vi "Arduino Microcontrollers.vi"   [LabVIEW 2011]
uses:
  _GlobalVariables&Libraries/ATV Program Global Variables.vi
  <vilib>/LabVIEW Interface for Arduino/LabVIEW Interface for Arduino.lvlib
types:
  T1 = cluster{"Arduino 1 VISA resource":refnum<visa-resource-name>, "Front Right Sonar Analog In Voltage":dbl, "Front Left Sonar Analog In Voltage":dbl, "Disable Arduino 1":bool}
  T2 = cluster{"Arduino 2 VISA resource":refnum<visa-resource-name>, "Front Center I2C Data":u8[], "Disable Arduino 2":bool, "Rear Left I2C Data":u8[], "Rear Right I2C Data":u8[]}
  T3 = typedef "LabVIEW Interface for Arduino.lvlib/Arduino Resource.ctl" = cluster{"VISA resource":refnum<visa-resource-name>, "Board Type":T4, "Connection Type":enum8{"USB / Serial"}, "Bytes Per Packet (15)":u8}
  T4 = typedef "LabVIEW Interface for Arduino.lvlib/Board Type.ctl" = enum16{"Uno", "Dimuelanove w/Atmega 328", "Mega 2560"}
  T5 = cluster{"Obstacle Detected":bool, "Drive Speed":string, "Steer Angle":string, "Left Object":bool, "Right Object":bool, "Center Object":bool, "Rear Left":bool, "Rear Right":bool}
  T6 = cluster{"End ATV Program":bool, "E-Stop":bool, "Save Logfile":bool, "Logfile Iteration Delay (ms)":u32, "Loop iteration time (ms)":u32, "Logfile Location":path, "Default GPS Navigation Path":path, "Computer":string, "Default GPS Boundary Path":path}
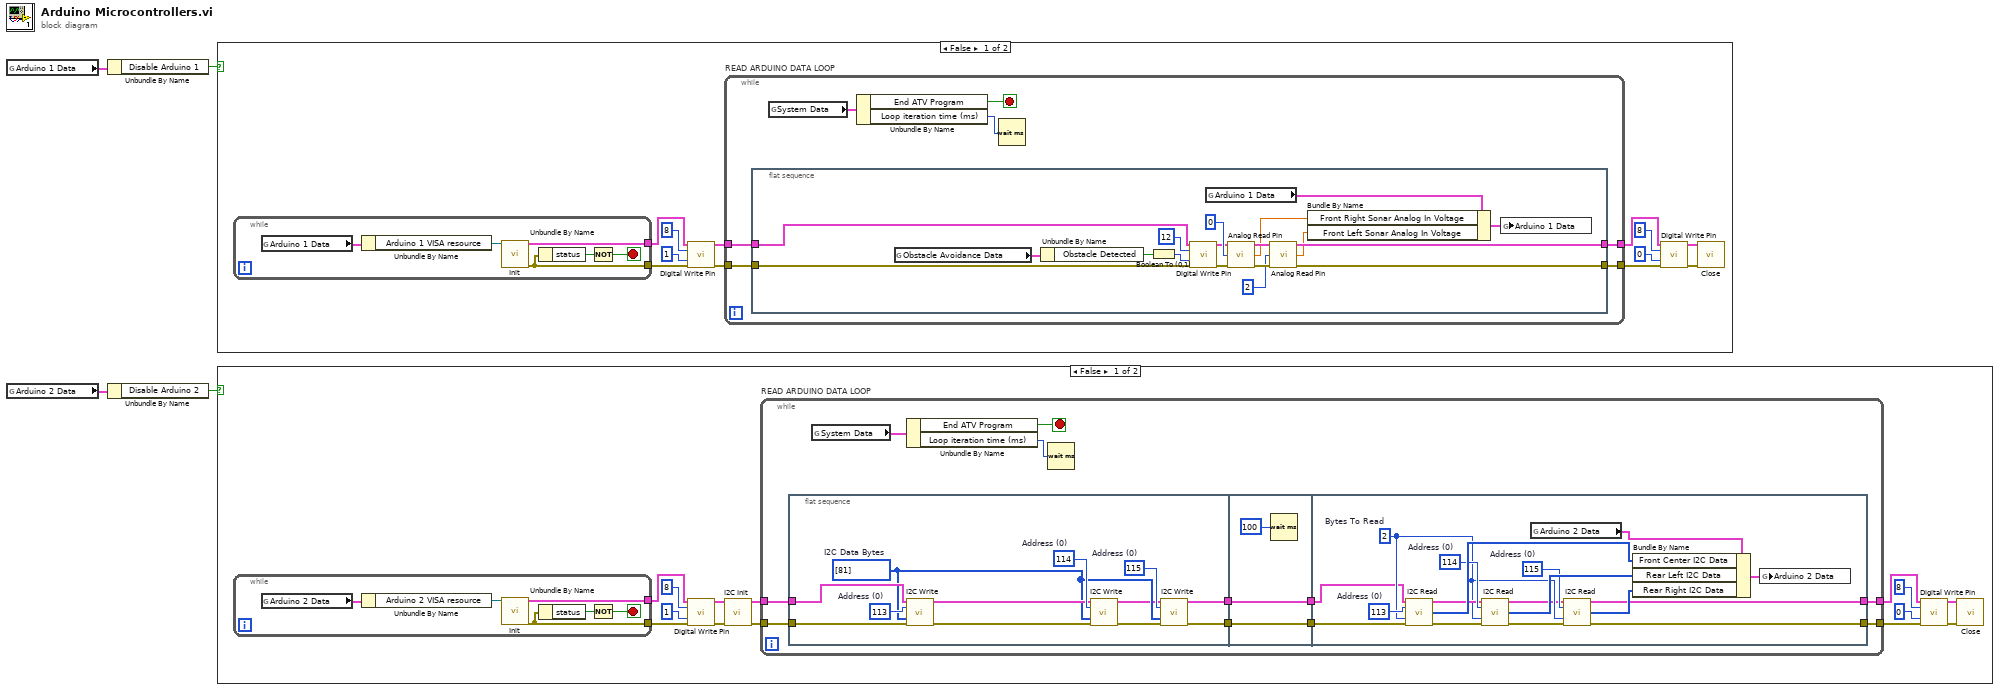
[diagram p0: block diagram]
diagram:
  n1 = global read "ATV Program Global Variables.vi" "Arduino 1 Data"() -> (w4:T1)
  n2 = global read "ATV Program Global Variables.vi" "Arduino 2 Data"() -> (w2:T2)
  n3 = Unbundle By Name(w4) -> ("Disable Arduino 1"=w3:bool)
  n4 = Unbundle By Name(w2) -> ("Disable Arduino 2"=w1:bool)
  n5 = case shown="False" w3 {
    frame False {
      n6 = while {
        tunnel: [w22] -> w16
        tunnel: [w21] -> w15
        stop <- w17 stop-if-true
        n7 = global read "ATV Program Global Variables.vi" "Arduino 1 Data"() -> (w20:T1)
        n8 = Unbundle By Name(w20) -> ("Arduino 1 VISA resource"=w19:refnum<visa-resource-name>)
        n9 = call <vilib>:"Init.vi"("VISA resource"=w19) -> ("Arduino Resource"=w22:T3, "error out"=w21:errorcluster)  [unwired: 17 in]
        n10 = Unbundle By Name(w21) -> ("status"=w18:bool)
        n11 = Not(x=w18) -> (.not. x?=w17:bool)
      }
      n12 = call <vilib>:"Digital Write Pin.vi"("Arduino Resource"=w16, "Digital I/O Pin (0)"=u8 8, "Value (0)"=u8 1, "error in"=w15) -> ("Arduino Resource"=w14:T3, "error out"=w13:errorcluster)  [unwired: 10 in]
      n13 = while "READ ARDUINO DATA LOOP" {
        tunnel: [w29] -> w10
        tunnel: [w28] -> w9
        tunnel: w14 -> [w24]
        tunnel: w13 -> [w23]
        stop <- w26 stop-if-true
        n14 = flat-sequence {
          tunnel: [w44] -> w28
          tunnel: [w45] -> w29
          tunnel: w24 -> [w35]
          tunnel: w23 -> [w34]
          frame #0 {
            n15 = global read "ATV Program Global Variables.vi" "Obstacle Avoidance Data"() -> (w31:T5)
            n16 = Unbundle By Name(w31) -> ("Obstacle Detected"=w30:bool)
            n17 = Boolean To (0,1)(Boolean=w30) -> (0, 1=w37:i16)
            n18 = call <vilib>:"Digital Write Pin.vi"("Arduino Resource"=w35, "Digital I/O Pin (0)"=u8 12, "Value (0)"=w37, "error in"=w34) -> ("Arduino Resource"=w33:T3, "error out"=w32:errorcluster)  [unwired: 10 in]
            n19 = global read "ATV Program Global Variables.vi" "Arduino 1 Data"() -> (w41:T1)
            n20 = call <vilib>:"Analog Read Pin.vi"("Arduino Resource"=w33, "Analog Input Pin (0)"=u8 0, "error in"=w32) -> ("Arduino Resource"=w47:T3, "Voltage"=w39:dbl, "error out"=w46:errorcluster)  [unwired: 10 in]
            n21 = call <vilib>:"Analog Read Pin.vi"("Arduino Resource"=w47, "Analog Input Pin (0)"=u8 2, "error in"=w46) -> ("Arduino Resource"=w45:T3, "Voltage"=w38:dbl, "error out"=w44:errorcluster)  [unwired: 10 in]
            n22 = Bundle By Name(cluster=w41, "Front Right Sonar Analog In Voltage"=w39, "Front Left Sonar Analog In Voltage"=w38) -> (w40:T1)
            n23 = global write "ATV Program Global Variables.vi" "Arduino 1 Data"(w40) -> ()
          }
        }
        n24 = global read "ATV Program Global Variables.vi" "System Data"() -> (w27:T6)
        n25 = Unbundle By Name(w27) -> ("End ATV Program"=w26:bool, "Loop iteration time (ms)"=w25:u32)
        n26 = Wait (ms)(milliseconds to wait=w25) -> ()  [unwired: 1 out]
      }
      n27 = call <vilib>:"Digital Write Pin.vi"("Arduino Resource"=w10, "Digital I/O Pin (0)"=u8 8, "Value (0)"=u8 0, "error in"=w9) -> ("Arduino Resource"=w8:T3, "error out"=w7:errorcluster)  [unwired: 10 in]
      n28 = call <vilib>:"Close.vi"("Arduino Resource"=w8, "error in"=w7) -> ()  [unwired: 13 in, 1 out]
    }
    frame True {
    }
  }
  n29 = case shown="False" w1 {
    frame False {
      n30 = while {
        tunnel: [w67] -> w59
        tunnel: [w66] -> w58
        stop <- w62 stop-if-true
        n31 = global read "ATV Program Global Variables.vi" "Arduino 2 Data"() -> (w65:T2)
        n32 = Unbundle By Name(w65) -> ("Arduino 2 VISA resource"=w64:refnum<visa-resource-name>)
        n33 = call <vilib>:"Init.vi"("VISA resource"=w64) -> ("Arduino Resource"=w67:T3, "error out"=w66:errorcluster)  [unwired: 17 in]
        n34 = Unbundle By Name(w66) -> ("status"=w63:bool)
        n35 = Not(x=w63) -> (.not. x?=w62:bool)
      }
      n36 = call <vilib>:"Digital Write Pin.vi"("Arduino Resource"=w59, "Digital I/O Pin (0)"=u8 8, "Value (0)"=u8 1, "error in"=w58) -> ("Arduino Resource"=w55:T3, "error out"=w54:errorcluster)  [unwired: 10 in]
      n37 = call <vilib>:"I2C Init.vi"("Arduino Resource"=w55, "error in"=w54) -> ("Arduino Resource"=w61:T3, "error out"=w60:errorcluster)  [unwired: 12 in]
      n38 = while "READ ARDUINO DATA LOOP" {
        tunnel: w61 -> [w75]
        tunnel: w60 -> [w74]
        tunnel: [w73] -> w48
        tunnel: [w72] -> w49
        stop <- w77 stop-if-true
        n39 = flat-sequence {
          tunnel: w75 -> [w89]
          tunnel: w74 -> [w88]
          tunnel: [w80] -> w70
          tunnel: [w79] -> w69
          tunnel: [w92] -> w71
          tunnel: w70 -> [w92]
          tunnel: w69 -> [w91]
          tunnel: [w91] -> w68
          tunnel: [w97] -> w72
          tunnel: [w96] -> w73
          tunnel: w71 -> [w95]
          tunnel: w68 -> [w94]
          frame #0 {
            w84 = u8 115  # Address (0)
            w87 = u8 114  # Address (0)
            w83 = u8[] [81]  # I2C Data Bytes
            w90 = u8 113  # Address (0)
            n40 = call <vilib>:"I2C Write.vi"("Arduino Resource"=w89, "Address (0)"=w90, "I2C Data Bytes"=w83, "error in"=w88) -> ("Arduino Resource"=w86:T3, "error out"=w85:errorcluster)  [unwired: 10 in]
            n41 = call <vilib>:"I2C Write.vi"("Arduino Resource"=w86, "Address (0)"=w87, "I2C Data Bytes"=w83, "error in"=w85) -> ("Arduino Resource"=w82:T3, "error out"=w81:errorcluster)  [unwired: 10 in]
            n42 = call <vilib>:"I2C Write.vi"("Arduino Resource"=w82, "Address (0)"=w84, "I2C Data Bytes"=w83, "error in"=w81) -> ("Arduino Resource"=w80:T3, "error out"=w79:errorcluster)  [unwired: 10 in]
          }
          frame #1 {
            n43 = Wait (ms)(milliseconds to wait=u32 100) -> ()  [unwired: 1 out]
          }
          frame #2 {
            w102 = u8 115  # Address (0)
            w106 = u8 114  # Address (0)
            w110 = u8 113  # Address (0)
            w101 = u8 2  # Bytes To Read
            n44 = call <vilib>:"I2C Read.vi"("Arduino Resource"=w95, "Address (0)"=w110, "Bytes To Read"=w101, "error in"=w94) -> ("Arduino Resource"=w105:T3, "I2C Data"=w108:u8[], "error out"=w104:errorcluster)  [unwired: 9 in]
            n45 = call <vilib>:"I2C Read.vi"("Arduino Resource"=w105, "Address (0)"=w106, "Bytes To Read"=w101, "error in"=w104) -> ("Arduino Resource"=w99:T3, "I2C Data"=w103:u8[], "error out"=w98:errorcluster)  [unwired: 9 in]
            n46 = global read "ATV Program Global Variables.vi" "Arduino 2 Data"() -> (w109:T2)
            n47 = call <vilib>:"I2C Read.vi"("Arduino Resource"=w99, "Address (0)"=w102, "Bytes To Read"=w101, "error in"=w98) -> ("Arduino Resource"=w97:T3, "I2C Data"=w100:u8[], "error out"=w96:errorcluster)  [unwired: 9 in]
            n48 = Bundle By Name(cluster=w109, "Front Center I2C Data"=w108, "Rear Left I2C Data"=w103, "Rear Right I2C Data"=w100) -> (w107:T2)
            n49 = global write "ATV Program Global Variables.vi" "Arduino 2 Data"(w107) -> ()
          }
        }
        n50 = global read "ATV Program Global Variables.vi" "System Data"() -> (w78:T6)
        n51 = Unbundle By Name(w78) -> ("End ATV Program"=w77:bool, "Loop iteration time (ms)"=w76:u32)
        n52 = Wait (ms)(milliseconds to wait=w76) -> ()  [unwired: 1 out]
      }
      n53 = call <vilib>:"Digital Write Pin.vi"("Arduino Resource"=w49, "Digital I/O Pin (0)"=u8 8, "Value (0)"=u8 0, "error in"=w48) -> ("Arduino Resource"=w51:T3, "error out"=w50:errorcluster)  [unwired: 10 in]
      n54 = call <vilib>:"Close.vi"("Arduino Resource"=w51, "error in"=w50) -> ()  [unwired: 13 in, 1 out]
    }
    frame True {
    }
  }
